vi "B field arrays.vi"() -> ()   [LabVIEW 2016]
panel:
  out "Waveform Graph 2":dbl[][](graph)
  out "Waveform Graph":i32[][](graph)
  in  "B fields":dbl[][](array[numeric])
  in  "Array":i32[][](array[numeric])
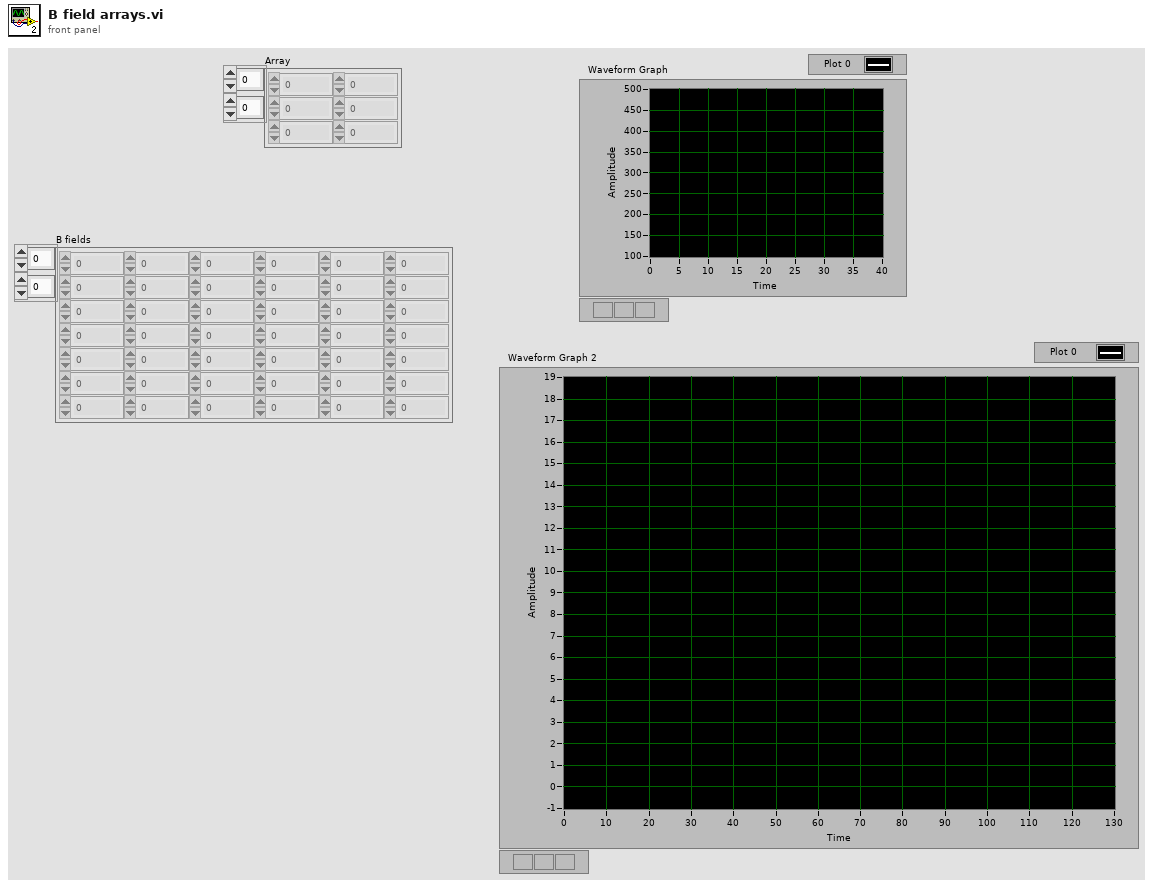
[diagram p1: front panel]
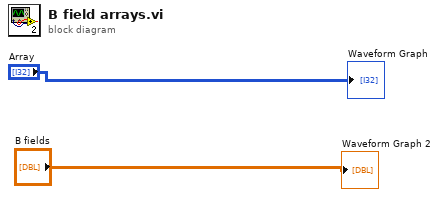
[diagram p0: block diagram]
diagram:
  "Waveform Graph" <- "Array"
  "Waveform Graph 2" <- "B fields"
